vi "Write I8.vi"(8 "error in (no error)":errorcluster, 10 "I8":i8, 11 "Event in":refnum<class "Event I8.lvclass">) -> (0 "error out":errorcluster, 3 "Event out":refnum<class "Event I8.lvclass">)   [LabVIEW 2017, in "Event Actors.lvlib" / "Event I8.lvclass"]
uses:
  Event I8.lvclass
  Event I8.lvclass/Event I8.ctl
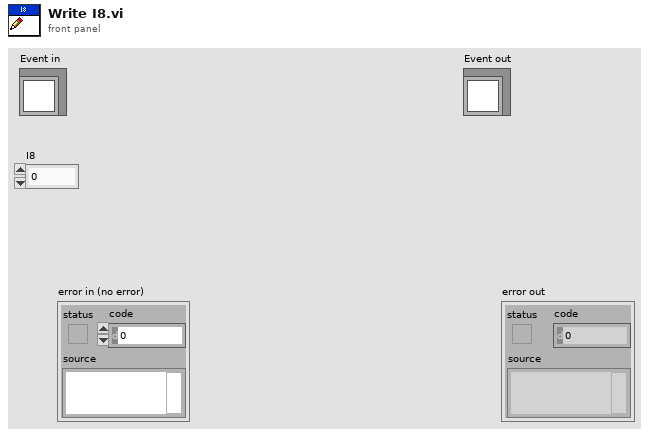
[diagram p1: front panel]
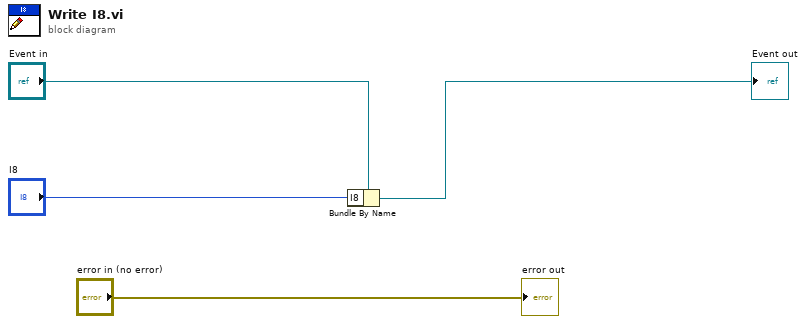
[diagram p0: block diagram]
diagram:
  n1 = Bundle By Name(cluster="Event in", "I8"="I8") -> (→"Event out":refnum<class "Event I8.lvclass">)
  "error out" <- "error in (no error)"
